vi "RT Driver VI.vi"(6 "Device Clock":string, 9 "Device Inputs FIFO":refnum<k33>, 10 "Device Outputs FIFO":refnum<k33>, 11 "Device Reference":T1 format="%.0x") -> ()   [LabVIEW 2016, in "UDP Transmit Engine.lvlib"]
uses:
  UDP Transmit Engine.lvlib
  <vilib>/NI Veristand/Custom Device API/Custom Device Item Ref.ctl
  <vilib>/NI Veristand/Custom Device API/Custom Device Channel Type.ctl
  <vilib>/NI Veristand/Custom Device API/Custom Device API.lvlib
  <vilib>/NI Veristand/Custom Device Tools/Custom Device Utility Library/Custom Device Utility Library.lvlib
panel:
  in  "Initialization Status Notifier":refnum<notifier>
  in  "Status Notifier":refnum<notifier>
  # "Custom Device Template\nv1.0"
  # "Use this template as a starting point for creating a custom device code module. The input controls shown here are specially named controls that the system will use to provide the device loop with data. The controls are not required for the device loop to run. For instance, if the device doesn't produce any output data, then you don't need the Device Outputs FIFO control. If you do use these controls, however, they need to have these exact names to be functional."
  # "The optional status notifier element is used to notify the RT engine of the last state of the custom device, and to indicate the device has completed execution. If this control is not used, a default No Error value is returned to the system when the device finishes execution.\n\nNote: This error state is not checked until the system shuts down. Use an output status channel to send more immediate status values to the system."
  # "This optional input can be used to send the VeriStand Engine the final status of the custom device initalization process. If this control exists on the custom device front panel, the VeriStand Engine will wait for a status update before starting up. If the custom device reports an error, that will abort the execution of the current configuration in the VeriStand Engine.\n\nThis control can be deleted if the custom device does not need to send the initialization status update."
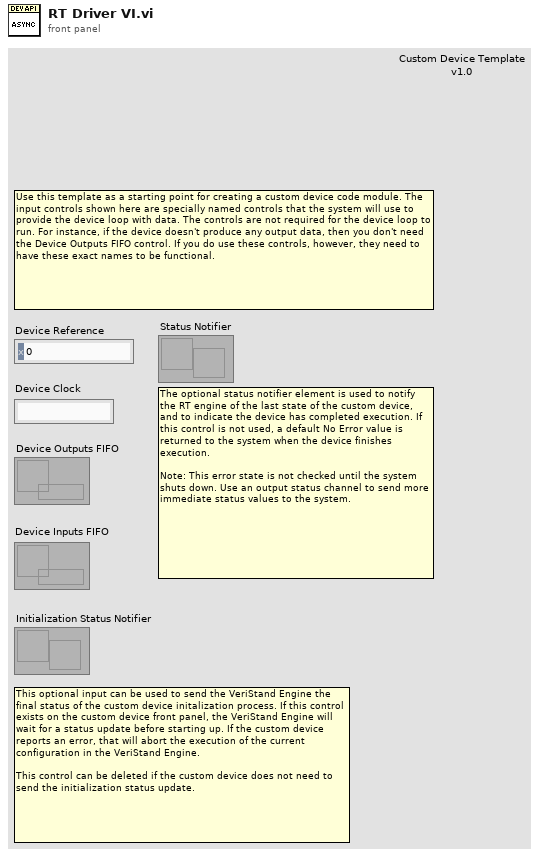
[diagram p1: front panel]
types:
  T1 = typedef "Custom Device API.lvlib/Custom Device Item Ref.ctl" = u64
  T2 = typedef "Custom Device API.lvlib/Custom Device Channel Type.ctl" = enum16{"Input", "Output"}
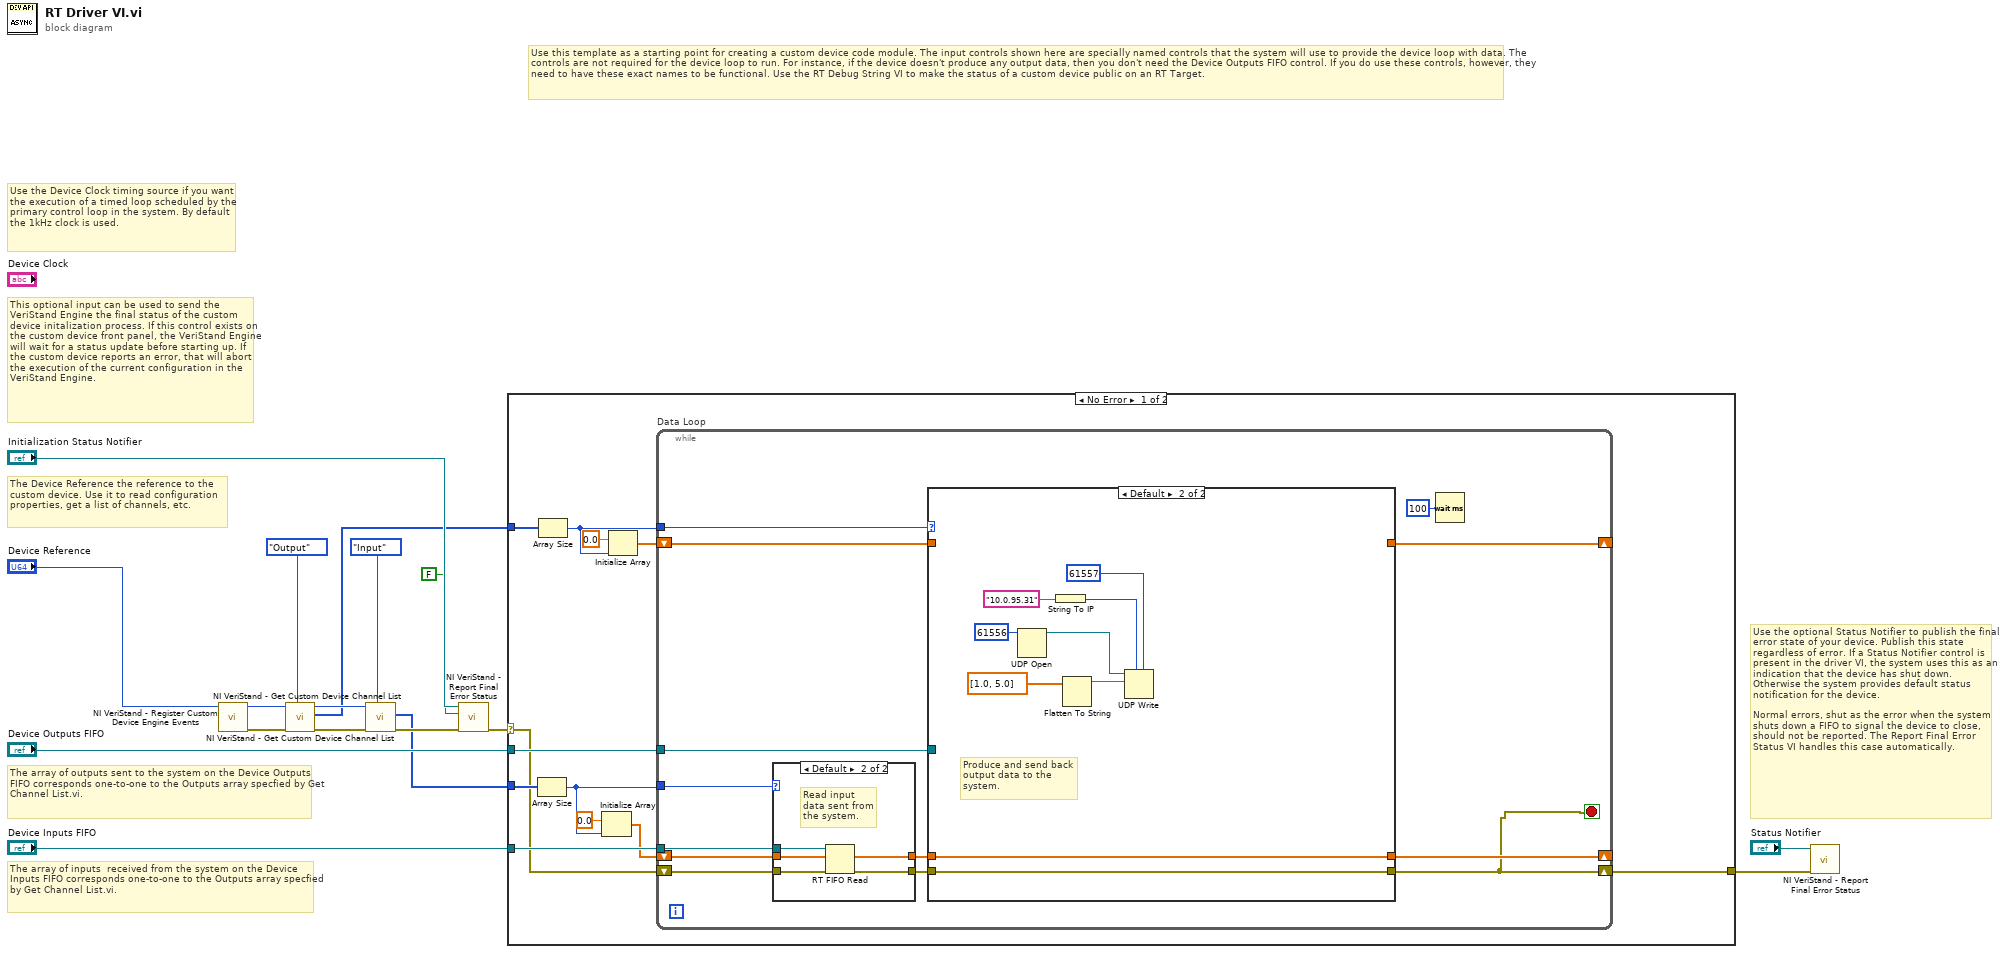
[diagram p0: block diagram]
diagram:
  # "This optional input can be used to send the VeriStand Engine the final status of the custom device initalization process. If this control exists on the custom device front panel, the VeriStand Engine will wait for a status update before starting up. If the custom device reports an error, that will abort the execution of the current configuration in the VeriStand Engine."
  # "The array of inputs  received from the system on the Device Inputs FIFO corresponds one-to-one to the Outputs array specfied by Get Channel List.vi."
  # "Use the optional Status Notifier to publish the final error state of your device. Publish this state regardless of error. If a Status Notifier control is present in the driver VI, the system uses this as an indication that the device has shut down. Otherwise the system provides default status notification for the device.\n\nNormal errors, shut as the error when the system shuts down a FIFO to signal the device to close, should not be reported. The Report Final Error Status VI handles this case automatically."
  # "The array of outputs sent to the system on the Device Outputs FIFO corresponds one-to-one to the Outputs array specfied by Get Channel List.vi."
  # "The Device Reference the reference to the custom device. Use it to read configuration properties, get a list of channels, etc."
  # "Use the Device Clock timing source if you want the execution of a timed loop scheduled by the primary control loop in the system. By default the 1kHz clock is used."
  # "Use this template as a starting point for creating a custom device code module. The input controls shown here are specially named controls that the system will use to provide the device loop with data. The controls are not required for the device loop to run. For instance, if the device doesn't produce any output data, then you don't need the Device Outputs FIFO control. If you do use these controls, however, they need to have these exact names to be functional. Use the RT Debug String VI to make the status of a custom device public on an RT Target."
  n1 = call <vilib>:"NI VeriStand - Register Custom Device Engine Events.vi"("Device Ref in"="Device Reference") -> ("error out"=w17:errorcluster, "Device Ref out"=w3:T1)  [unwired: 8 in, 1 out]
  n2 = call <vilib>:"NI VeriStand - Get Custom Device Channel List.vi"("Channel Type"=Custom_Device_Channel_Type."Output", "error in (no error)"=w17, "Device Ref in"=w3) -> ("error out"=w10:errorcluster, "Specified Channel Ref List"=w7:T1[], "Device Ref out"=w11:T1)  [unwired: 6 out]
  n3 = call <vilib>:"NI VeriStand - Get Custom Device Channel List.vi"("Channel Type"=Custom_Device_Channel_Type."Input", "error in (no error)"=w10, "Device Ref in"=w11) -> ("error out"=w16:errorcluster, "Specified Channel Ref List"=w8:T1[])  [unwired: 7 out]
  n4 = call <vilib>:"NI VeriStand - Report Final Error Status.vi"("error in (no error)"=w16, "Filter FIFO & Shutdown Errors (T)"=FALSE ("Filter FIFO Errors (T)"), "Status Notifier"="Initialization Status Notifier") -> ("error out"=w2:errorcluster)  [unwired: 8 out]
  n5 = case shown="No Error" w2 {
    selector: w2 -> [w19 w62]
    tunnel: "Device Outputs FIFO" -> [w29 _]
    tunnel: "Device Inputs FIFO" -> [w28 _]
    tunnel: w8 -> [w22 _]
    tunnel: w7 -> [w21 _]
    tunnel: [w18 w62] -> w5
    frame No Error {
      n6 = Array Size(array=w22) -> (size(s)=w20:i32)
      n7 = Array Size(array=w21) -> (size(s)=w23:i32)
      n8 = Initialize Array(0.0 ("element"), w20) -> (w24:dbl[])
      n9 = Initialize Array(0.0 ("element"), w23) -> (w25:dbl[])
      n10 = while "Data Loop" {
        shift-right: [w40] -> _
        shift-left: w24 -> [w41]
        shift-right: [w30] -> w18
        shift-left: w19 -> [w42]
        shift-right: [w38] -> _
        shift-left: w25 -> [w39]
        tunnel: w23 -> [w35]
        tunnel: w29 -> [w37]
        tunnel: w28 -> [w36]
        tunnel: w20 -> [w34]
        stop <- w30 stop-if-true
        n11 = case shown="Default" w34 {
          tunnel: w36 -> [_ w61]
          tunnel: w41 -> [w56 w60]
          tunnel: [w56 w59] -> w33
          tunnel: [w55 w58] -> w32
          tunnel: w42 -> [w55 w57]
          frame 0 {
            # "No inputs to read\nfrom system. Inputs FIFO not created in this case, so don't write to it."
          }
          frame Default {
            # "Read input data sent from the system."
            n12 = RT FIFO Read(0:w61, 1:w60, 3:w57) -> (9:w59:dbl[], 11:w58:errorcluster)  [unwired: 4 out]
          }
        }
        n13 = case shown="Default" w35 {
          tunnel: w37 -> [_ _]
          tunnel: w39 -> [w45 _]
          tunnel: w33 -> [w44 w54]
          tunnel: w32 -> [w43 w47]
          tunnel: [w43 w47] -> w30
          tunnel: [w45 _] -> w38
          tunnel: [w44 w54] -> w40
          frame 0 {
            # "No outputs to write to system. The Device Outputs FIFO is never created in this case, so don't write to it."
          }
          frame Default {
            # "Produce and send back output data to the system."
            n14 = UDP Open(11:u16 61556 ("port")) -> (port=w50:refnum<k16>)  [unwired: 4 in, 2 out]
            n15 = String To IP(1:"10.0.95.31") -> (0:w51:u32)
            n16 = Flatten To String(anything=dbl[] [1.0, 5.0]) -> (data string=w48:string)  [unwired: 3 in, 2 out]
            n17 = UDP Write(address=w51, port or service name=u16 61557, connection ID=w50, data in=w48) -> ()  [unwired: 2 in, 2 out]
          }
        }
        n18 = Wait (ms)(milliseconds to wait=u32 100) -> ()  [unwired: 1 out]
      }
    }
    frame Error {
    }
  }
  n19 = call <vilib>:"NI VeriStand - Report Final Error Status.vi"("error in (no error)"=w5, "Status Notifier"="Status Notifier") -> ()  [unwired: 1 in, 9 out]
